vi "updateArrays_pos_names_status-BellaAlpha.vi"(0 "name/data 2":string[][](array[string]), 5 "#ofChannels":i32=7, 7 "max channels":i32=10) -> (4 "pos":T2[](array[typedef]), 6 "Names":string[](array[string]), 8 "Description":string[](array[string]), 10 "Status":u32[](array[colorbox]), 15 "Mode":T1[](array[typedef]))   [LabVIEW 2013]
uses:
  Device Drivers/FilterWheels/posTypDef.ctl
  Device Drivers/FilterWheels/ModeTypDEf.ctl
panel:
  out "Numeric 2":i32
  out "Numeric":i32
  out "Position":string[](array[string])
  out "Array 3":string[][](array[string])
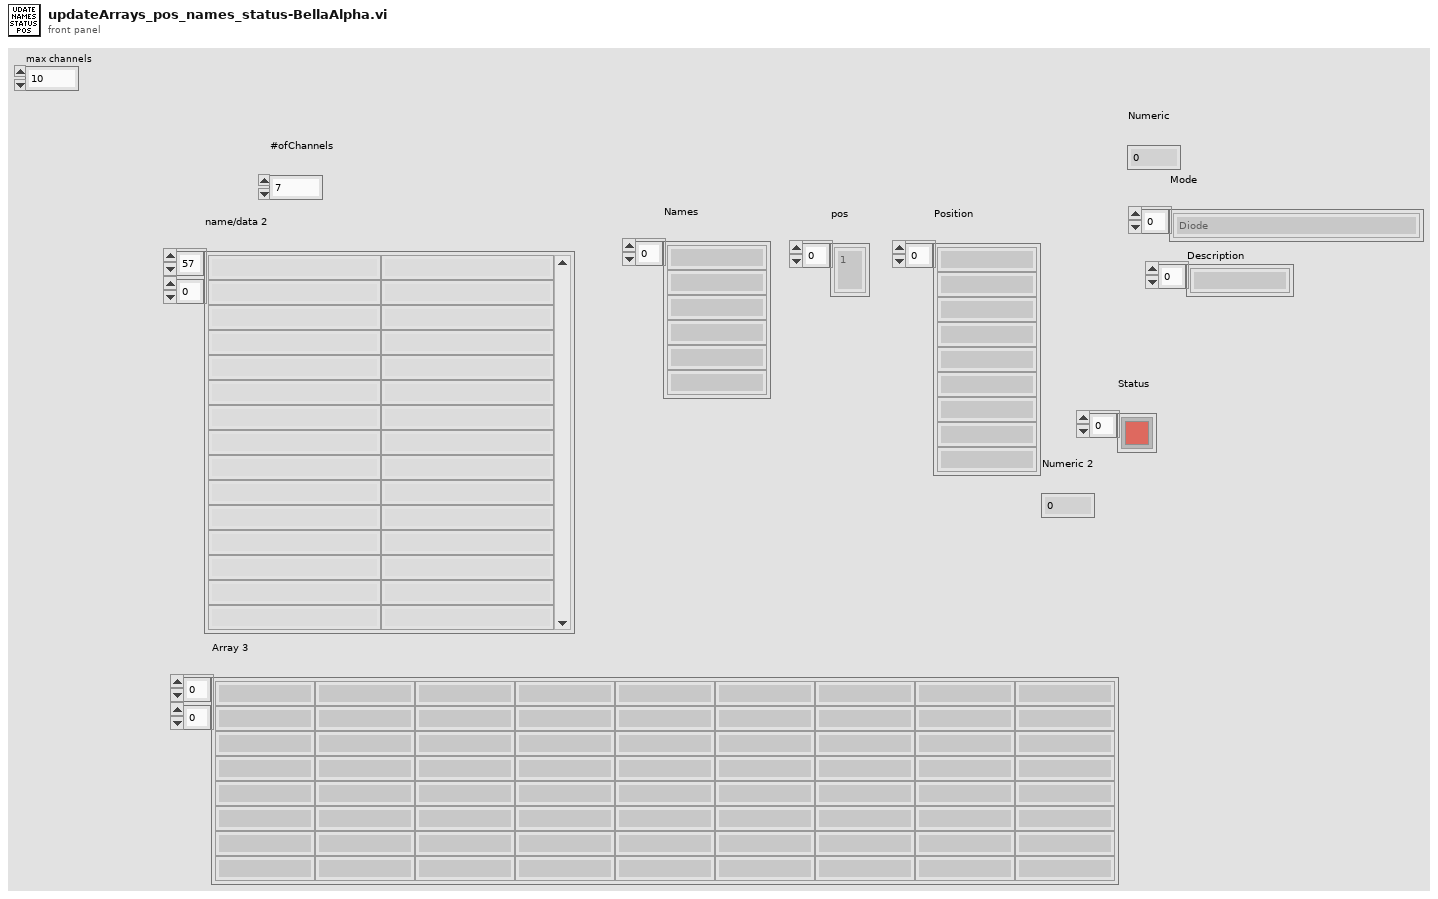
[diagram p1: front panel]
types:
  T1 = typedef "ModeTypDEf.ctl" = enum16{"Diode", "Low Power", "High Power", "undefined"}
  T2 = typedef "posTypDef.ctl" = enum16{"1", "2", "3", "4", "5", "6"}
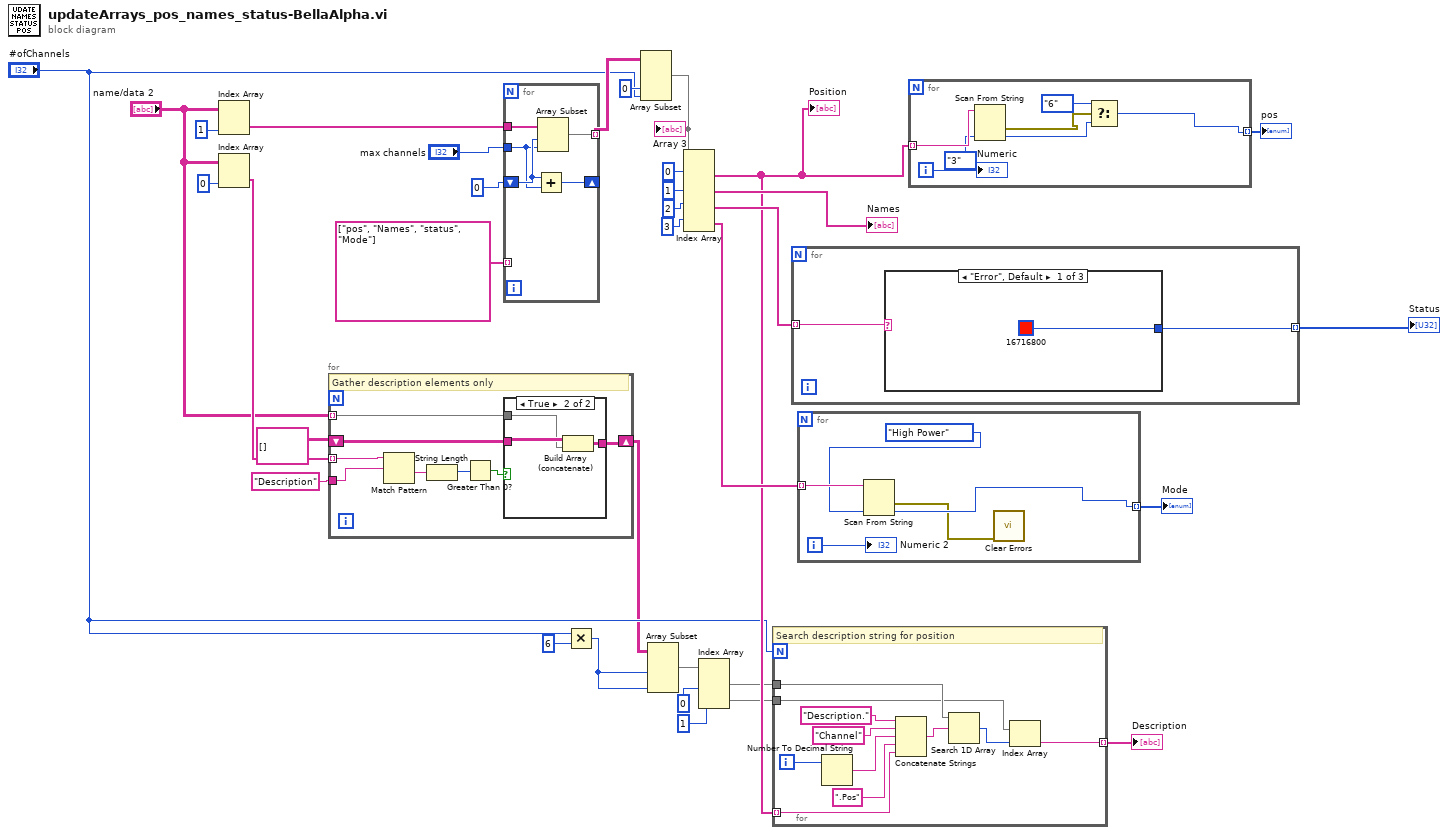
[diagram p0: block diagram]
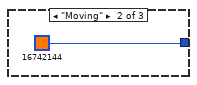
[diagram p2: hidden frame]
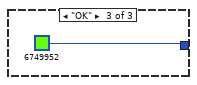
[diagram p3: hidden frame]
diagram:
  n1 = Index Array(array="name/data 2", index (col)=1 ("disabled index (col)")) -> (element=w16:string[])  [unwired: 1 in]
  n2 = Index Array(array="name/data 2", index (col)=0 ("disabled index (col)")) -> (element=w15:string[])  [unwired: 1 in]
  n3 = for {
    shift-right: [w36] -> w8
    shift-left: string[][] [] ("subarray") -> [w38]
    tunnel: "Description" -> [w42]
    tunnel: w15 -> [w37] mode=indexing
    tunnel: "name/data 2" -> [w35] mode=indexing
    # "Gather description elements only"
    n4 = Match Pattern(string=w37, regular expression=w42) -> (after substring=w41:string)  [unwired: 1 in, 3 out]
    n5 = String Length(string=w41) -> (length=w39:i32)
    n6 = Greater Than 0?(x=w39) -> (x > 0?=w40:bool)
    n7 = case shown="True" w40 {
      tunnel: w38 -> [w43 w46]
      tunnel: [w43 w45] -> w36
      tunnel: w35 -> [_ w44]
      frame False {
      }
      frame True {
        n8 = Build Array (concatenate)(w46, w44) -> (w45:string[][])
      }
    }
  }
  n9 = for {
    tunnel: string[] ["pos", "Names", "status", "Mode"] -> [_] mode=indexing
    tunnel: w16 -> [w48]
    shift-right: [w49] -> _
    shift-left: 0 ("offset past match") -> [w51]
    tunnel: "max channels" -> [w50]
    tunnel: [w47] -> w22 mode=indexing
    n10 = Add(x=w51, y=w50) -> (x+y=w49:i32)
    n11 = Array Subset(array=w48, index=w51, length=w50) -> (w47:string[])
  }
  n12 = Multiply(x="#ofChannels", y=6) -> (x*y=w11:i32)
  n13 = Array Subset(array=w22, index (col)=0 ("index"), length (col)="#ofChannels") -> (w20:string[][])  [unwired: 2 in]
  "Array 3" <- w20
  n14 = Array Subset(array=w8, length (row)=w11, length (col)=w11) -> (w5:string[][])  [unwired: 2 in]
  n15 = Index Array(array=w20, index (row) #1=0 ("index (row)"), index (row) #2=1 ("index (row)"), index (row) #3=2 ("index (row)"), index (row) #4=3 ("index (row)")) -> (element #1=w10:string[], element #2=→"Names":string[], element #3=w27:string[], element #4=w19:string[])  [unwired: 4 in]
  "Position" <- w10
  n16 = Index Array(array=w5, index (col) #1=0 ("disabled index (col)"), index (col) #2=1 ("index (col)")) -> (element #1=w7:string[], element #2=w3:string[])  [unwired: 2 in]
  n17 = for {
    N: "#ofChannels" -> [_]
    tunnel: w10 -> [w52] mode=indexing
    tunnel: w7 -> [w57]
    tunnel: w3 -> [w55]
    tunnel: [w53] -> w2 mode=indexing
    i -> [w60]
    # "Search description string for position"
    n18 = Number To Decimal String(number=w60) -> (decimal integer string=w59:string)  [unwired: 1 in]
    n19 = Concatenate Strings("Description.", "Channel" ("string"), w59, ".Pos" ("string"), w52) -> (w56:string)
    n20 = Search 1D Array(1D array=w57, element=w56) -> (index of element=w54:i32)  [unwired: 1 in]
    n21 = Index Array(array=w55, index=w54) -> (element=w53:string)
  }
  "Description" <- w2
  n22 = for {
    tunnel: w27 -> [w64] mode=indexing
    tunnel: [w63] -> w24 mode=indexing
    n23 = case shown="\"Error\", Default" w64 {
      tunnel: [u32 16716800 u32 16742144 u32 6749952] -> w63
      frame "Error", Default {
      }
      frame "Moving" {
      }
      frame "OK" {
      }
    }
  }
  "Status" <- w24
  n24 = for {
    tunnel: w19 -> [w72] mode=indexing
    tunnel: [w69] -> w25 mode=indexing
    i -> [w71]
    n25 = Scan From String(input string=w72, default 1=ModeTypDEf."High Power" ("Mode")) -> (error out=w68:errorcluster, output 1=w69:T1)  [unwired: 3 in, 2 out]
    n26 = call <vilib>:"Clear Errors.vi"("error in (no error)"=w68) -> ()  [unwired: 6 in, 1 out]
    "Numeric 2" <- w71
  }
  "Mode" <- w25
  n27 = for {
    tunnel: w10 -> [w79] mode=indexing
    tunnel: [w74] -> w1 mode=indexing
    i -> [w77]
    n28 = Scan From String(input string=w79, default 1=posTypDef."3" ("Channel1")) -> (error out=w76:errorcluster, output 1=w75:T2)  [unwired: 3 in, 2 out]
    n29 = Select(t=posTypDef."6", s=w76, f=w75) -> (s? t:f=w74:T2)
    "Numeric" <- w77
  }
  "pos" <- w1
